vi "Gestione lista esiti.vi"() -> ()   [LabVIEW 2019]
panel:
  in  "COLLEGAMENTO":u16(ring)=1 items=["GRUPPO ELETTROGENO", "ALTERNATORE", "GENERICO", "MOTORE C.A.", "MOTORE EEX", "MOTORE C.C.", "POMPA", "TRASFORMATORE"]
  in  "SVUOTA":bool
  in  "elimina selezionato":bool
  in  "Refresh Button":bool
  in  "SALVA COME":bool
  in  "FILE GESTIONE ESITI":string(combo)
  in  "SALVA NOMI ESITI":bool
  in  "GESTIONE ESITI":T1
  # "Nota: per eliminare un elemento dalle liste tendine\ncliccarci sopra col tasto destro e scegliere \"Delete element\""
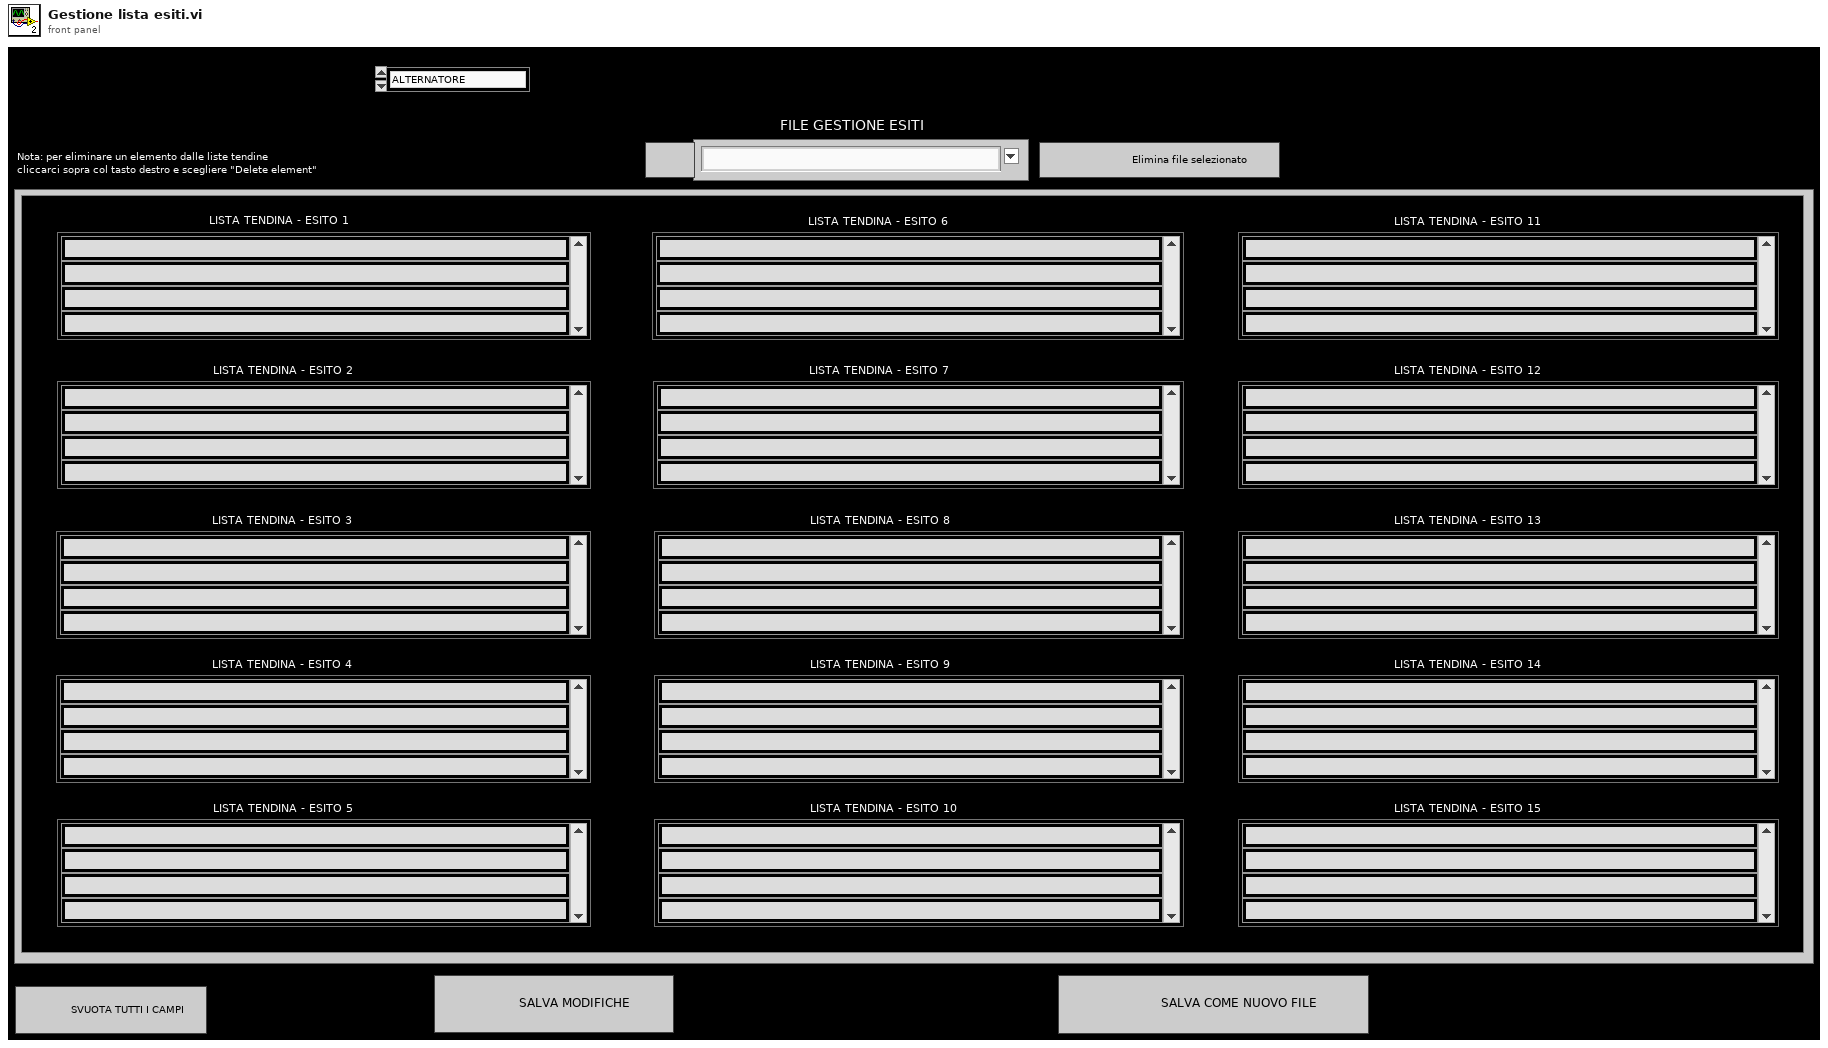
[diagram p1: front panel]
types:
  T1 = cluster{"LISTA TENDINA - ESITO 1":string[], "LISTA TENDINA - ESITO 2":string[], "LISTA TENDINA - ESITO 3":string[], "LISTA TENDINA - ESITO 4":string[], "LISTA TENDINA - ESITO 5":string[], "LISTA TENDINA - ESITO 6":string[], "LISTA TENDINA - ESITO 7":string[], "LISTA TENDINA - ESITO 8":string[], "LISTA TENDINA - ESITO 9":string[], "LISTA TENDINA - ESITO 10":string[], "LISTA TENDINA - ESITO 11":string[], "LISTA TENDINA - ESITO 12":string[], "LISTA TENDINA - ESITO 13":string[], "LISTA TENDINA - ESITO 14":string[], "LISTA TENDINA - ESITO 15":string[]}
  T2 = enum16{"open", "replace", "create", "open or create", "replace or create", "replace or create with confirmation"}
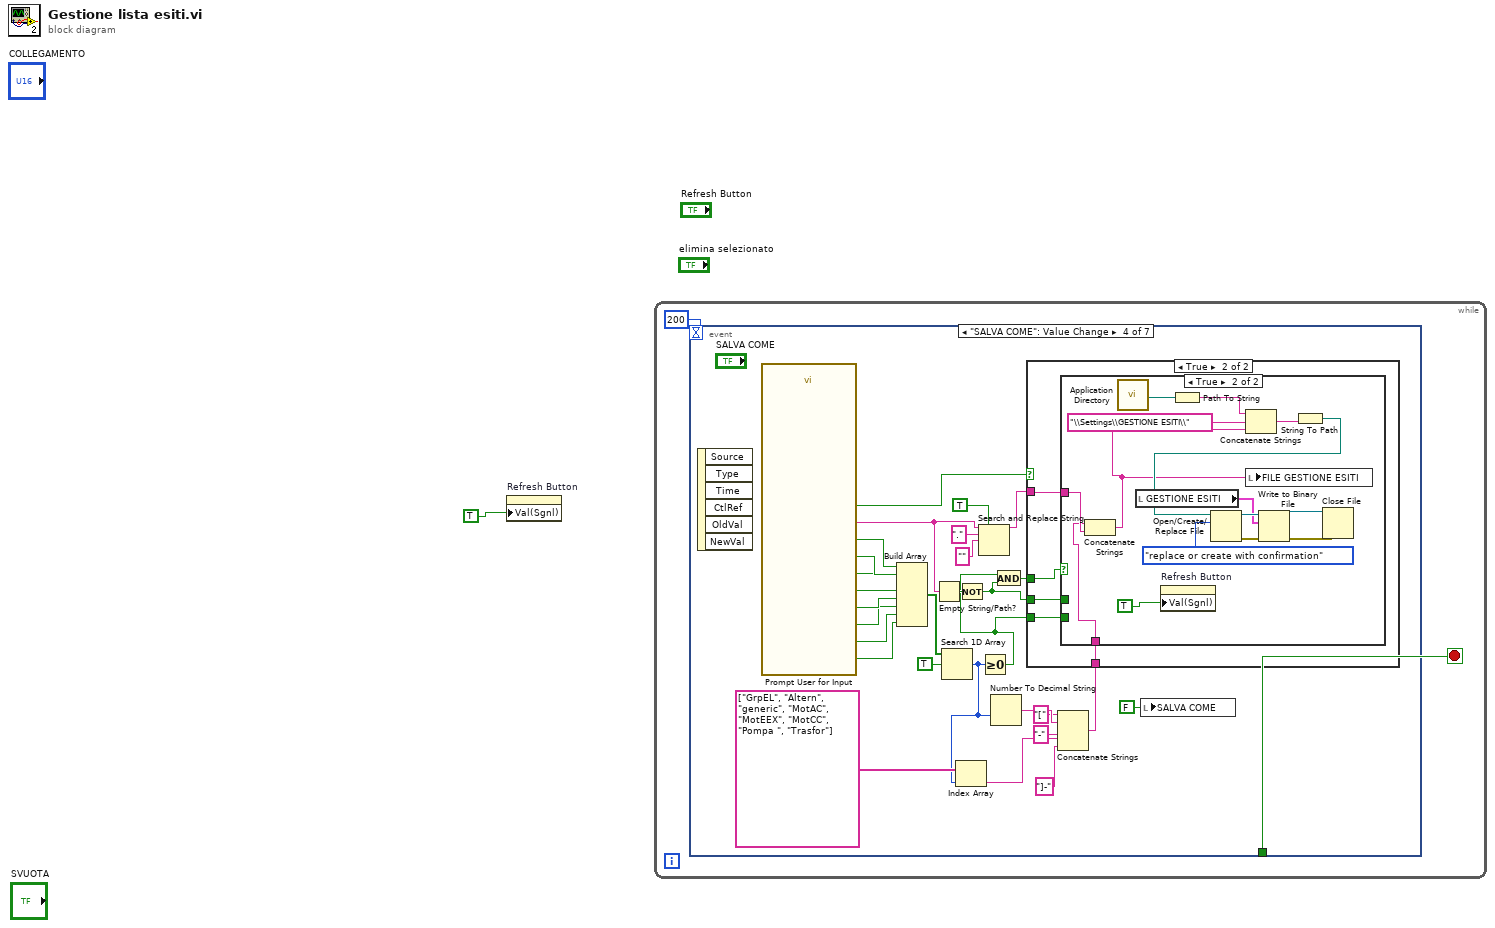
[diagram p0: block diagram]
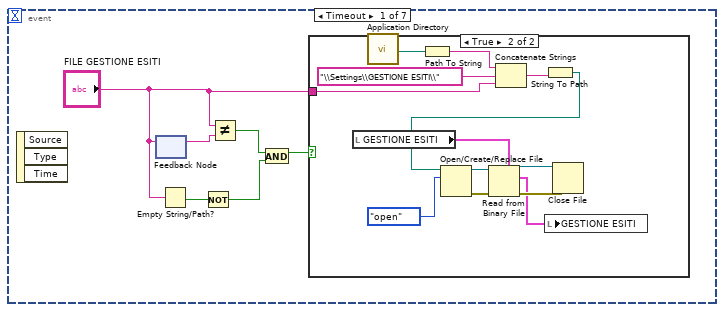
[diagram p2: hidden frame]
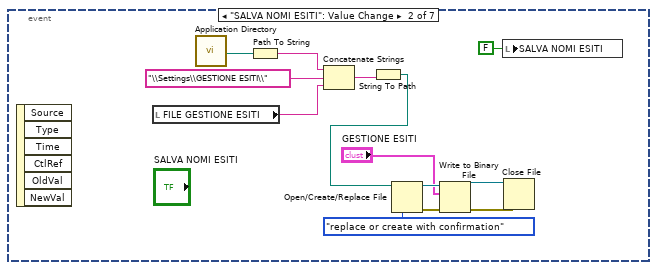
[diagram p4: hidden frame]
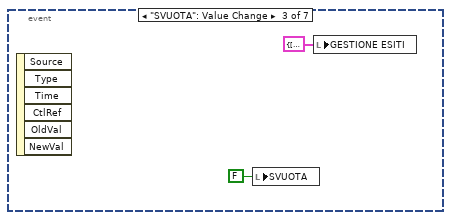
[diagram p5: hidden frame]
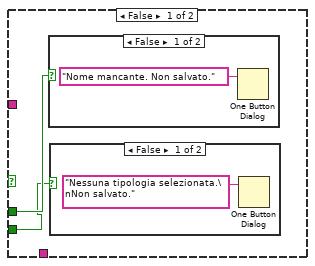
[diagram p7: hidden frame]
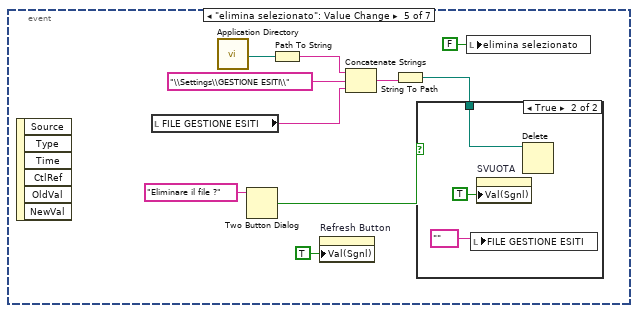
[diagram p10: hidden frame]
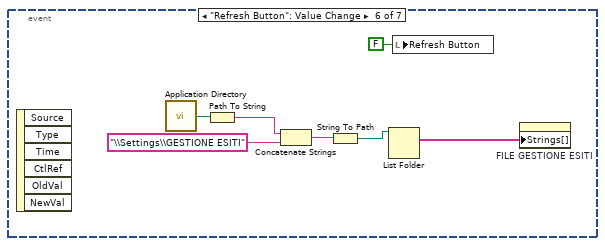
[diagram p12: hidden frame]
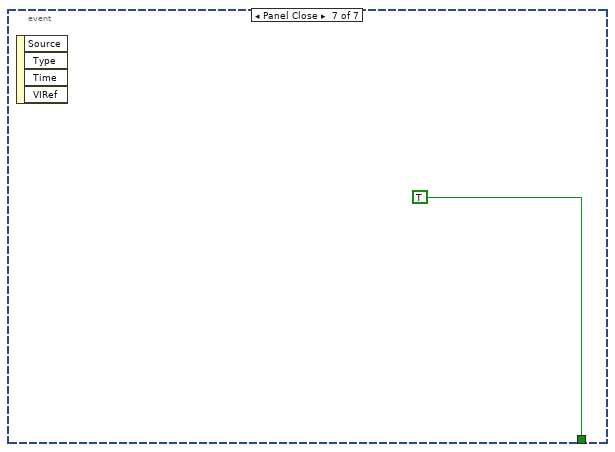
[diagram p13: hidden frame]
diagram:
  n1 = property on="Refresh Button" class="Bool (strict)"("Val(Sgnl)"=TRUE) -> ()  [unwired: 2 in, 2 out]
  n2 = while {
    stop <- w3 stop-if-true
    n3 = event shown="[3] \"SALVA COME\": Value Change" {
      selector: _ -> [_ _ _ _ _ _ _]
      dyn-events: _ -> [_ _ _ _ _ _ _]
      timeout: 200 -> [_ _ _ _ _ _ _]
      tunnel: [_ _ _ _ _ _ TRUE] -> w3
      event Timeout {
        n4 = event-data() -> ()  [unwired: 1 in, 3 out]
        n5 = feedback-in #1("FILE GESTIONE ESITI") -> ()
        n6 = feedback #1() -> (w9:string)  [unwired: 1 in]
        n7 = Empty String/Path?(string/path="FILE GESTIONE ESITI") -> (empty?=w5:bool)
        n8 = Not(x=w5) -> (.not. x?=w4:bool)
        n9 = Not Equal?(x="FILE GESTIONE ESITI", y=w9) -> (x != y?=w8:bool)
        n10 = And(x=w8, y=w4) -> (x .and. y?=w6:bool)
        n11 = case shown="True" w6 {
          tunnel: "FILE GESTIONE ESITI" -> [_ w18]
          frame False {
          }
          frame True {
            n12 = local read "GESTIONE ESITI"() -> (w11:T1)
            n13 = call <vilib>:"Application Directory.vi"() -> ("Application Directory"=w22:path)
            n14 = Path To String(path=w22) -> (string=w20:string)
            n15 = Concatenate Strings(w20, "\\Settings\\GESTIONE ESITI\\" ("string"), w18) -> (w21:string)
            n16 = String To Path(string=w21) -> (path=w13:path)
            n17 = Open/Create/Replace File(file path (use dialog)=w13, operation (0:open)=T2."open") -> (refnum out=w16:refnum<file>, error out=w17:errorcluster)  [unwired: 4 in, 1 out]
            n18 = Read from Binary File(5:w11, 8:w17, 11:w16) -> (0:w15:errorcluster, 2:w10:T1, 3:w14:refnum<file>)  [unwired: 3 in, 1 out]
            n19 = local write "GESTIONE ESITI"(w10) -> ()
            n20 = Close File(refnum=w14, error in=w15) -> ()  [unwired: 2 out]
          }
        }
      }
      event "SALVA NOMI ESITI": Value Change {
        n21 = event-data() -> ()  [unwired: 1 in, 6 out]
        n22 = local read "FILE GESTIONE ESITI"() -> (w24:string)
        n23 = call <vilib>:"Application Directory.vi"() -> ("Application Directory"=w29:path)
        n24 = Path To String(path=w29) -> (string=w27:string)
        n25 = Concatenate Strings(w27, "\\Settings\\GESTIONE ESITI\\" ("string"), w24) -> (w28:string)
        n26 = String To Path(string=w28) -> (path=w25:path)
        n27 = Open/Create/Replace File(file path (use dialog)=w25, operation (0:open)=T2."replace or create with confirmation") -> (refnum out=w34:refnum<file>, error out=w35:errorcluster)  [unwired: 4 in, 1 out]
        n28 = Write to Binary File(file (use dialog)=w34, data="GESTIONE ESITI", error in=w35) -> (refnum out=w32:refnum<file>, error out=w33:errorcluster)  [unwired: 3 in, 1 out]
        n29 = local write "SALVA NOMI ESITI"(FALSE ("SALVA NOMI ESITI")) -> ()
        n30 = Close File(refnum=w32, error in=w33) -> ()  [unwired: 2 out]
      }
      event "SVUOTA": Value Change {
        n31 = event-data() -> ()  [unwired: 1 in, 6 out]
        n32 = local write "SVUOTA"(FALSE ("SVUOTA")) -> ()
        n33 = local write "GESTIONE ESITI"(T1 {"LISTA TENDINA - ESITO 1"=[], "LISTA TENDINA - ESITO 2"=[], "LISTA TENDINA - ESITO 3"=[], "LISTA TENDINA - ESITO 4"=[], "LISTA TENDINA - ESITO 5"=[], "LISTA TENDINA - ESITO 6"=[], "LISTA TENDINA - ESITO 7"=[], "LISTA TENDINA - ESITO 8"=[], "LISTA TENDINA - ESITO 9"=[], "LISTA TENDINA - ESITO 10"=[], "LISTA TENDINA - ESITO 11"=[], "LISTA TENDINA - ESITO 12"=[], "LISTA TENDINA - ESITO 13"=[], "LISTA TENDINA - ESITO 14"=[], "LISTA TENDINA - ESITO 15"=[]} ("GESTIONE ESITI")) -> ()
      }
      event "SALVA COME": Value Change {
        n34 = event-data() -> ()  [unwired: 1 in, 6 out]
        n35 = call "Prompt User for Input"() -> ("TRASFORMATORE"=w53:bool, "POMPA"=w54:bool, "MOTORE CC"=w55:bool, "MOTORE EEX"=w56:bool, "MOTORE AC"=w57:bool, "GENERICO"=w58:bool, "ALTERNATORE"=w59:bool, "GRUPPO ELETTROGENO"=w60:bool, "Nome"=w50:string, "OK"=w66:bool)  [unwired: 9 in, 1 out]
        n36 = Build Array(w60, w59, w58, w57, w56, w55, w54, w53) -> (w52:bool[])
        n37 = Empty String/Path?(string/path=w50) -> (empty?=w48:bool)
        n38 = Search 1D Array(1D array=w52, element=TRUE) -> (index of element=w39:i32)  [unwired: 1 in]
        n39 = Index Array(array=string[] ["GrpEL", "Altern", "generic", "MotAC", "MotEEX", "MotCC", "Pompa ", "Trasfor"], index=w39) -> (element=w38:string)
        n40 = Not(x=w48) -> (.not. x?=w47:bool)
        n41 = Search and Replace String(replace all?=TRUE ("replace all? (F)"), input string=w50, search string=".", replace string="" ("replace string (\"\")")) -> (result string=w64:string)  [unwired: 4 in, 3 out]
        n42 = Greater Or Equal To 0?(x=w39) -> (x >= 0?=w46:bool)
        n43 = Number To Decimal String(number=w39) -> (decimal integer string=w45:string)  [unwired: 1 in]
        n44 = And(x=w46, y=w47) -> (x .and. y?=w49:bool)
        n45 = Concatenate Strings("[" ("string"), w45, "-" ("string"), w38, "]-" ("string")) -> (w43:string)
        n46 = case shown="True" w66 {
          tunnel: w64 -> [_ w71]
          tunnel: w49 -> [_ w70]
          tunnel: w47 -> [_ w69]
          tunnel: w46 -> [_ w68]
          tunnel: w43 -> [_ w67]
          frame False {
          }
          frame True {
            n47 = case shown="True" w70 {
              tunnel: w71 -> [_ w77]
              tunnel: w69 -> [w73 _]
              tunnel: w68 -> [w72 _]
              tunnel: w67 -> [_ w76]
              frame False {
                n48 = case shown="False" w73 {
                  frame False {
                    n49 = One Button Dialog(message="Nome mancante. Non salvato.") -> ()  [unwired: 1 in, 1 out]
                  }
                  frame True {
                  }
                }
                n50 = case shown="False" w72 {
                  frame False {
                    n51 = One Button Dialog(message="Nessuna tipologia selezionata.\nNon salvato.") -> ()  [unwired: 1 in, 1 out]
                  }
                  frame True {
                  }
                }
              }
              frame True {
                n52 = Concatenate Strings(w76, w77) -> (w78:string)
                n53 = call <vilib>:"Application Directory.vi"() -> ("Application Directory"=w90:path)
                n54 = local read "GESTIONE ESITI"() -> (w80:T1)
                n55 = property on="Refresh Button" class="Bool (strict)"("Val(Sgnl)"=TRUE) -> ()  [unwired: 2 in, 2 out]
                n56 = Path To String(path=w90) -> (string=w88:string)
                n57 = Concatenate Strings(w88, "\\Settings\\GESTIONE ESITI\\" ("string"), w78) -> (w89:string)
                n58 = local write "FILE GESTIONE ESITI"(w78) -> ()
                n59 = String To Path(string=w89) -> (path=w81:path)
                n60 = Open/Create/Replace File(file path (use dialog)=w81, operation (0:open)=T2."replace or create with confirmation") -> (refnum out=w85:refnum<file>, error out=w86:errorcluster)  [unwired: 4 in, 1 out]
                n61 = Write to Binary File(file (use dialog)=w85, data=w80, error in=w86) -> (refnum out=w83:refnum<file>, error out=w84:errorcluster)  [unwired: 3 in, 1 out]
                n62 = Close File(refnum=w83, error in=w84) -> ()  [unwired: 2 out]
              }
            }
          }
        }
        n63 = local write "SALVA COME"(FALSE ("SALVA COME")) -> ()
      }
      event "elimina selezionato": Value Change {
        n64 = event-data() -> ()  [unwired: 1 in, 6 out]
        n65 = local read "FILE GESTIONE ESITI"() -> (w96:string)
        n66 = call <vilib>:"Application Directory.vi"() -> ("Application Directory"=w100:path)
        n67 = Two Button Dialog(message="Eliminare il file ?") -> (T button?=w94:bool)  [unwired: 2 in]
        n68 = Path To String(path=w100) -> (string=w98:string)
        n69 = property on="Refresh Button" class="Bool (strict)"("Val(Sgnl)"=TRUE ("Value (Signaling)")) -> ()  [unwired: 2 in, 2 out]
        n70 = Concatenate Strings(w98, "\\Settings\\GESTIONE ESITI\\" ("string"), w96) -> (w99:string)
        n71 = String To Path(string=w99) -> (path=w95:path)
        n72 = case shown="True" w94 {
          tunnel: w95 -> [_ w103]
          frame False {
          }
          frame True {
            n73 = local write "FILE GESTIONE ESITI"("" ("FILE GESTIONE ESITI")) -> ()
            n74 = property on="SVUOTA" class="Bool (strict)"("Val(Sgnl)"=TRUE ("Value (Signaling)")) -> ()  [unwired: 2 in, 2 out]
            n75 = Delete(path (use dialog)=w103) -> ()  [unwired: 4 in, 3 out]
          }
        }
        n76 = local write "elimina selezionato"(FALSE ("elimina selezionato")) -> ()
      }
      event "Refresh Button": Value Change {
        n77 = event-data() -> ()  [unwired: 1 in, 6 out]
        n78 = call <vilib>:"Application Directory.vi"() -> ("Application Directory"=w109:path)
        n79 = Path To String(path=w109) -> (string=w110:string)
        n80 = Concatenate Strings(w110, "\\Settings\\GESTIONE ESITI" ("string")) -> (w108:string)
        n81 = String To Path(string=w108) -> (path=w106:path)
        n82 = List Folder(path=w106) -> (filenames=w105:string[])  [unwired: 3 in, 3 out]
        n83 = local write "Refresh Button"(FALSE ("Refresh Button")) -> ()
        n84 = property on="FILE GESTIONE ESITI" class="CmbBox"("Strings[]"=w105) -> ()  [unwired: 2 in, 2 out]
      }
      event Panel Close {
        n85 = event-data() -> ()  [unwired: 1 in, 4 out]
      }
    }
  }
